vi "test_generic.vi"() -> ()   [LabVIEW 2010, in "GenericStimulator.lvclass"]
uses:
  GenericStimulator.lvclass
  main/labview_source/type_definitions/clusters/controls_refs.ctl
  common/classes/GenericComponent/GenericComponent/GenericComponent.lvclass
  common/classes/GenericToplevelComponent/GenericToplevelComponent/common_trigger_enum.ctl
  common/classes/GenericToplevelComponent/GenericToplevelComponent/GenericToplevelComponent.lvclass
panel:
  in  "sweep button":bool
  in  "create button":bool
  in  "stop":bool
  # "Test Stimulator"
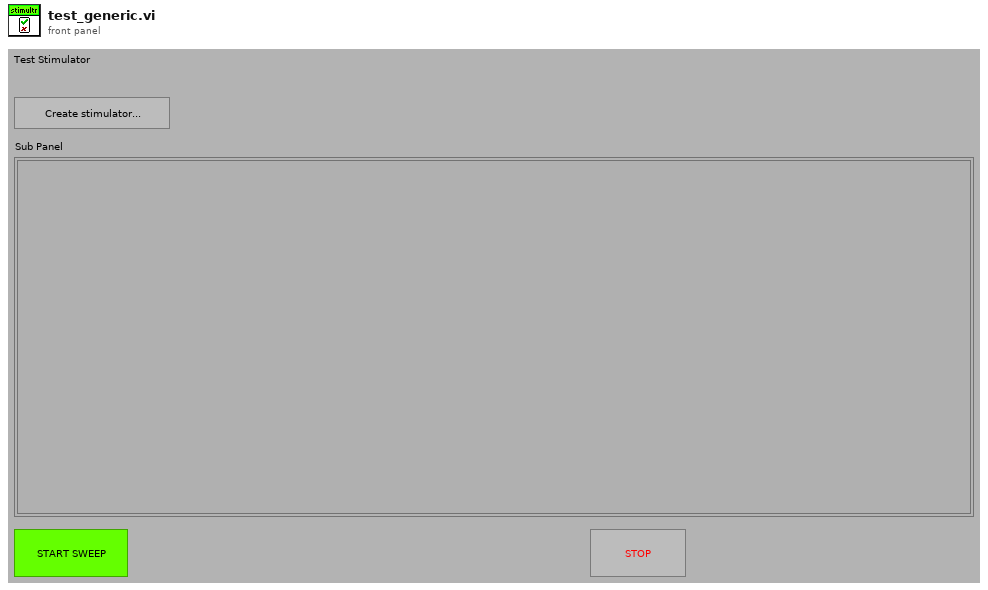
[diagram p1: front panel]
types:
  T1 = typedef "controls_refs.ctl" = cluster{"scan start button":refnum<vi>, "tabs":cluster{"main":refnum<vi>, "settings":refnum<vi>}, "subpanels":cluster{"imagingMode":refnum<vi>, "scanHead":refnum<vi>, "display":refnum<vi>, "experimentController":refnum<vi>, "instrument":refnum<vi>, "stage":refnum<vi>, "stimulator":refnum<vi>, "dataCollection":refnum<vi>, "analyser":refnum<vi>, "daq":refnum<vi>, "imageAssembler":refnum<vi>}, "drop-downs":cluster{"run mode":refnum<vi>, "imagingMode":refnum<vi>, "experimentalController":refnum<vi>, "objective":refnum<vi>}, "status lights":cluster{"experimentController":refnum<vi>, "imagingMode":refnum<vi>, "scanHead":refnum<vi>, "daq":refnum<vi>, "imageAssembler":refnum<vi>, "dataCollection":refnum<vi>, "display":refnum<vi>, "analyser":refnum<vi>, "stage":refnum<vi>, "stimulator":refnum<vi>, "instrument":refnum<vi>}, "message":refnum<vi>, "stimulator enabled?":refnum<vi>, "saving":cluster{"data folder path":refnum<vi>, "file base name":refnum<vi>, "notebook":refnum<vi>}, "progress bar":refnum<vi>, "update icon":refnum<vi>, "title":refnum<vi>, "main vi":refnum<vi>, "user":refnum<vi>, "exit_button":refnum<vi>, "CPU usage %":refnum<vi>}
  T2 = typedef "GenericToplevelComponent.lvclass/common_trigger_enum.ctl" = enum16{"NULL", "initialise", "terminate", "fetch command", "fetch data", "attach observer", "register as observer", "detach observer", "acknowledge", "start", "stop", "sweep started", "sweep stopped", "experiment started", "experiment stopped"}
  T3 = typedef "XComponentSpecification.xctl/data.ctl" = cluster{"class path":string, "configuration":string, "label":string, "settings name":string}
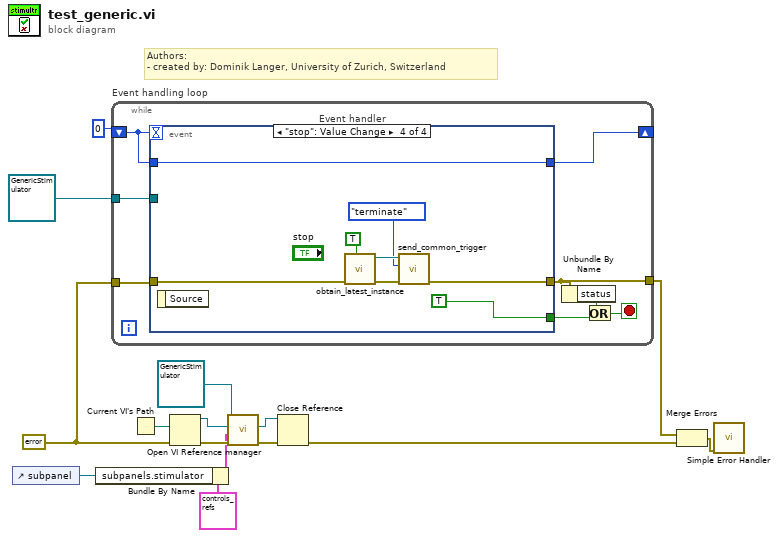
[diagram p0: block diagram]
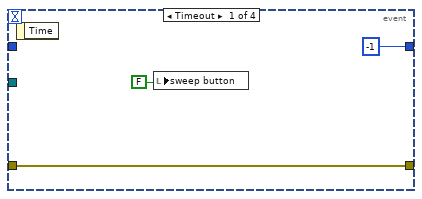
[diagram p2: hidden frame]
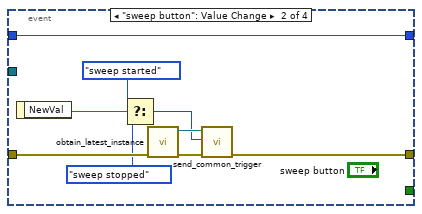
[diagram p3: hidden frame]
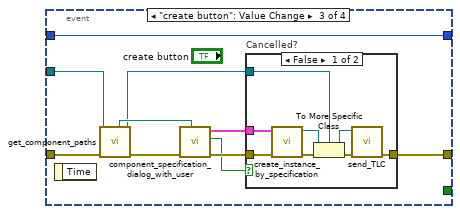
[diagram p4: hidden frame]
diagram:
  w10 = errorcluster {"status"=FALSE, "code"=0, "source"=""} ("error in (no error)")
  # "Authors: \n- created by: Dominik Langer, University of Zurich, Switzerland"
  n1 = control-ref of="subpanel"() -> (w12:refnum<vi>)
  n2 = Bundle By Name(cluster=T1 {"scan start button"=refnum, "tabs"={"main"=refnum, "settings"=refnum}, "subpanels"={"imagingMode"=refnum, "scanHead"=refnum, "display"=refnum, "experimentController"=refnum, "instrument"=refnum, "stage"=refnum, "stimulator"=refnum, "dataCollection"=refnum, "analyser"=refnum, "daq"=refnum, "imageAssembler"=refnum}, "drop-downs"={"run mode"=refnum, "imagingMode"=refnum, "experimentalController"=refnum, "objective"=refnum}, "status lights"={"experimentController"=refnum, "imagingMode"=refnum, "scanHead"=refnum, "daq"=refnum, "imageAssembler"=refnum, "dataCollection"=refnum, "display"=refnum, "analyser"=refnum, "stage"=refnum, "stimulator"=refnum, "instrument"=refnum}, "message"=refnum, "stimulator enabled?"=refnum, "saving"={"data folder path"=refnum, "file base name"=refnum, "notebook"=refnum}, "progress bar"=refnum, "update icon"=refnum, "title"=refnum, "main vi"=refnum, "user"=refnum, "exit_button"=refnum, "CPU usage %"=refnum} ("control references"), "subpanels.stimulator"=w12) -> (w2:T1)
  n3 = while "Event handling loop" {
    shift-right: [w21] -> _
    shift-left: 0 -> [w22]
    tunnel: refnum<class "GenericStimulator.lvclass"> refnum ("GenericStimulator.lvclass") -> [w20]
    tunnel: w10 -> [w23]
    tunnel: [w19] -> w14
    stop <- w16 stop-if-true
    n4 = event "Event handler" shown="[3] \"stop\": Value Change" {
      selector: _ -> [_ _ _ _]
      dyn-events: _ -> [_ _ _ _]
      timeout: w22 -> [_ _ _ _]
      tunnel: w23 -> [w24 w34 w39 w57]
      tunnel: w22 -> [_ w35 w45 w62]
      tunnel: [-1 w35 w45 w62] -> w21
      tunnel: [w24 w33 w44 w56] -> w19
      tunnel: [_ _ _ TRUE] -> w17
      tunnel: w20 -> [_ _ w41 _]
      event Timeout {
        n5 = event-data() -> ()  [unwired: 2 out]
        n6 = local write "sweep button"(FALSE) -> ()
      }
      event "sweep button": Value Change {
        n7 = event-data() -> ("NewVal"=w30:bool)  [unwired: 1 out]
        n8 = Select(t=common_trigger_enum."sweep started" ("trigger"), s=w30, f=common_trigger_enum."sweep stopped") -> (s? t:f=w28:T2)
        n9 = call "obtain_latest_instance.vi"("error in (no error)"=w34) -> ("error out"=w31:errorcluster, "GenericStimulator out"=w32:refnum<class "GenericStimulator.lvclass">)  [unwired: 1 in, 8 out]
        n10 = call-dynamic "send_common_trigger.vi"("error in (no error)"=w31, "trigger"=w28, "GenericToplevelComponent in"=w32) -> ("error out"=w33:errorcluster)  [unwired: 6 in, 2 out]
      }
      event "create button": Value Change {
        n11 = event-data() -> ()  [unwired: 2 out]
        n12 = call-dynamic "get_component_paths.vi"("error in (no error)"=w39, "GenericComponent in"=w41) -> ("error out"=w43:errorcluster, "GenericComponent out"=w40:refnum<class "GenericStimulator.lvclass">, "component type directory"=w42:path)  [unwired: 4 in, 3 out]
        n13 = call "component_specification_dialog_with_user.vi"("start path"=w42, "error in (no error)"=w43) -> ("error out"=w38:errorcluster, "cancelled?"=w37:bool, "component specification out"=w36:T3)  [unwired: 7 in]
        n14 = case "Cancelled?" shown="False" w37 {
          tunnel: [w53 w54] -> w44
          tunnel: w40 -> [w52 _]
          tunnel: w38 -> [w51 w54]
          tunnel: w36 -> [w46 _]
          frame False {
            n15 = call "create_instance_by_specification.vi"("error in (no error)"=w51, "component specification"=w46) -> ("error out"=w50:errorcluster, "GenericPlugin out"=w49:refnum<class "GenericComponent.lvclass">)  [unwired: 7 in, 1 out]
            n16 = To More Specific Class(target class=w52, reference=w49, error in=w50) -> (specific class reference=w47:refnum<class "GenericStimulator.lvclass">, error out=w48:errorcluster)
            n17 = call-dynamic "send_TLC.vi"("error in (no error)"=w48, "GenericToplevelComponent in"=w47) -> ("error out"=w53:errorcluster)  [unwired: 9 out]
          }
          frame True {
          }
        }
      }
      event "stop": Value Change {
        n18 = event-data() -> ()  [unwired: 2 out]
        n19 = call "obtain_latest_instance.vi"("quick, but maybe outdated?"=TRUE, "error in (no error)"=w57) -> ("error out"=w59:errorcluster, "GenericStimulator out"=w60:refnum<class "GenericStimulator.lvclass">)  [unwired: 8 out]
        n20 = call-dynamic "send_common_trigger.vi"("error in (no error)"=w59, "trigger"=common_trigger_enum."terminate", "GenericToplevelComponent in"=w60) -> ("error out"=w56:errorcluster)  [unwired: 6 in, 2 out]
      }
    }
    n21 = Unbundle By Name(w19) -> ("status"=w18:bool)
    n22 = Or(x=w18, y=w17) -> (x .or. y?=w16:bool)
  }
  n23 = Current VI's Path() -> (path=w9:path)
  n24 = Open VI Reference(vi path=w9, error in (no error)=w10) -> (vi reference=w3:refnum<vi>, error out=w6:errorcluster)  [unwired: 4 in]
  n25 = call-dynamic "manager.vi"("error in (no error)"=w6, "control references"=w2, "top-level VI ref in"=w3, "GenericToplevelComponent in"=refnum<class "GenericStimulator.lvclass"> refnum ("GenericStimulator.lvclass")) -> ("error out"=w5:errorcluster, "top-level VI ref out"=w1:refnum<vi>)  [unwired: 5 in, 1 out]
  n26 = Close Reference(reference=w1, error in (no error)=w5) -> (error out=w11:errorcluster)
  n27 = Merge Errors(w14, w11) -> (w15:errorcluster)
  n28 = call <vilib>:"Simple Error Handler.vi"("error in (no error)"=w15) -> ()  [unwired: 1 in, 8 out]
